vi "TEST1.vi"() -> ()   [LabVIEW 2018]
panel:
  in  "stop":bool
  in  "VOLTS\nOUT":dbl format="%#_3g"
  out "VOLTS\nIN":dbl format="%#_3g"
  in  "SWITCH\nC":bool
  in  "SWITCH\nB":bool
  in  "SWITCH\nA":bool
  out "LED\n2":bool
  out "LED\n1":bool
  out "LED\n0":bool
  # "DIGITAL INPUTS AND OUTPUTS"
  # "ANALOG INPUTS AND OUTPUTS"
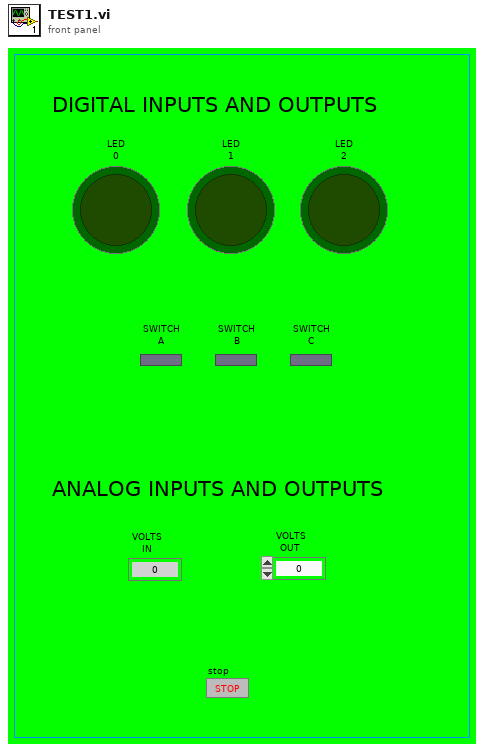
[diagram p1: front panel]
types:
  T1 = cluster{"data[0]":bool, "data[1]":bool, "data[2]":bool, "data[3]":bool, "data[4]":bool, "data[5]":bool, "data[6]":bool, "data[7]":bool, "data[8]":bool}
  T2 = cluster{"SWITCH\nA":bool, "SWITCH\nB":bool, "SWITCH\nC":bool}
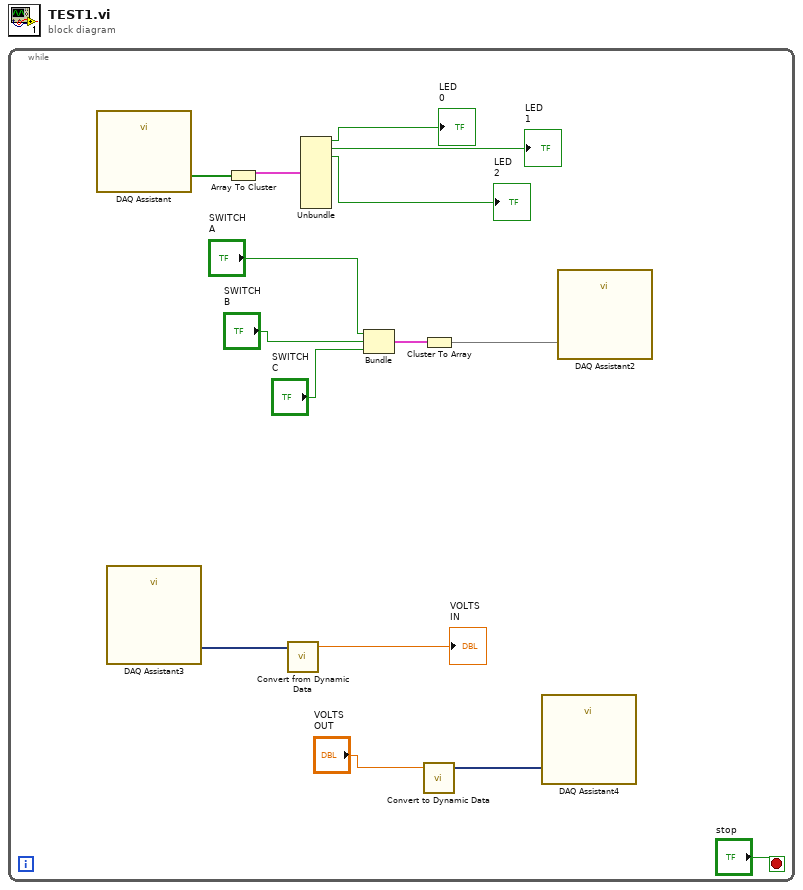
[diagram p0: block diagram]
diagram:
  n1 = while {
    stop <- "stop" stop-if-true
    n2 = call "DAQ Assistant"() -> ("data"=w15:bool[])  [unwired: 17 in, 2 out]
    n3 = call "DAQ Assistant3"() -> ("data"=w4:dynamicdata)  [unwired: 17 in, 2 out]
    n4 = Array To Cluster(array=w15) -> (cluster=w14:T1)
    n5 = call "Convert from Dynamic Data"("Dynamic Data Type"=w4) -> ("Scalar"=→"VOLTS\nIN":dbl)  [unwired: 3 in]
    n6 = Unbundle(w14) -> ("data[0]"=→"LED\n0":bool, "data[1]"=→"LED\n1":bool, "data[2]"=→"LED\n2":bool)  [unwired: 6 out]
    n7 = Bundle("SWITCH\nA"="SWITCH\nA", "SWITCH\nB"="SWITCH\nB", "SWITCH\nC"="SWITCH\nC") -> (w8:T2)  [unwired: 1 in]
    n8 = Cluster To Array(cluster=w8) -> (array=w9:bool[])
    n9 = call "Convert to Dynamic Data"("Double"="VOLTS\nOUT") -> ("Dynamic Data Type"=w1:dynamicdata)  [unwired: 3 in]
    n10 = call "DAQ Assistant4"("data"=w1) -> ()  [unwired: 17 in, 2 out]
    n11 = call "DAQ Assistant2"("data"=w9) -> ()  [unwired: 17 in, 2 out]
  }
